vi "_Remote Prepare Mass Range.vi"(9 "Run Mode":T1, 10 "Fixed Mass (amu)":dbl, 11 "GUI Mass Ranges":T5[](array[typedef]) {"Res" items=["High/High", "Medium/Medium", "Low/Low", "High/Medium", "High/Low", "Medium/High", "Medium/Low", "Low/High", "Low/Medium"]}) -> (0 "Steps":i32[](array[numeric]), 1 "Dwell (ms)":dbl[](array[numeric]), 2 "Mass":dbl[](array[numeric]), 3 "Cycle Time (ms)":dbl, 4 "Init Q2 Mass":i32, 6 "Init Q1 Mass":i32, 7 "RT Mass Ranges":T2[](array[typedef]) {"Resolution Type" items=["High/High", "Medium/Medium", "Low/Low", "High/Medium", "High/Low", "Medium/High", "Medium/Low", "Low/High", "Low/Medium"]})   [LabVIEW 2015]
uses:
  Type/_Mass Range Property.ctl
  Type/_Mass Range Parameters.ctl
  Type/_RT Res Type.ctl
  Type/_RT Mass Range.ctl
  Type/_RT Active Ch.ctl
  Type/_Run Mode.ctl
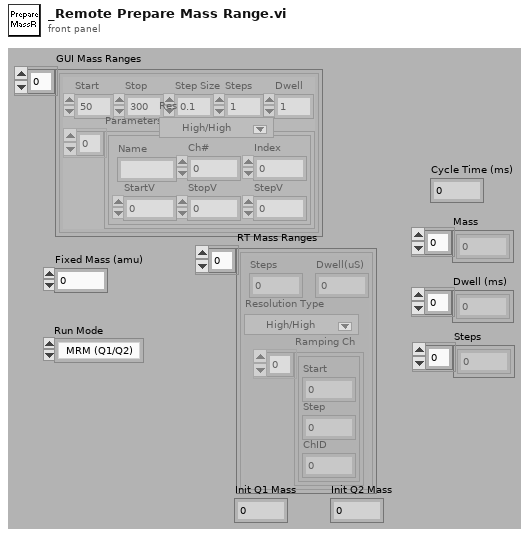
[diagram p1: front panel]
types:
  T1 = typedef "_Run Mode.ctl" = enum16{"MRM (Q1/Q2)", "Q1 Scan", "Q1 SRM", "Q2 Scan", "Q2 SRM", "Product Scan", "Precursor Scan", "Neutral Loss", "Neutral Gain"}
  T2 = typedef "_RT Mass Range.ctl" = cluster{"Steps":i32, "Dwell(uS)":i32, "Resolution Type":T3, "Ramping Ch":T4[]}
  T3 = typedef "_RT Res Type.ctl" = u16
  T4 = typedef "_RT Active Ch.ctl" = cluster{"Start":i32, "Step":i32, "ChID":i32}
  T5 = typedef "_Mass Range Property.ctl" = cluster{"Start":dbl, "Stop":dbl, "Step Size":dbl, "Steps":i32, "Dwell":dbl, "Parameters":T6[], "Res":T3}
  T6 = typedef "_Mass Range Parameters.ctl" = cluster{"Name":string, "Ch#":u8, "StartV":dbl, "StopV":dbl, "StepV":dbl, "Index":u8}
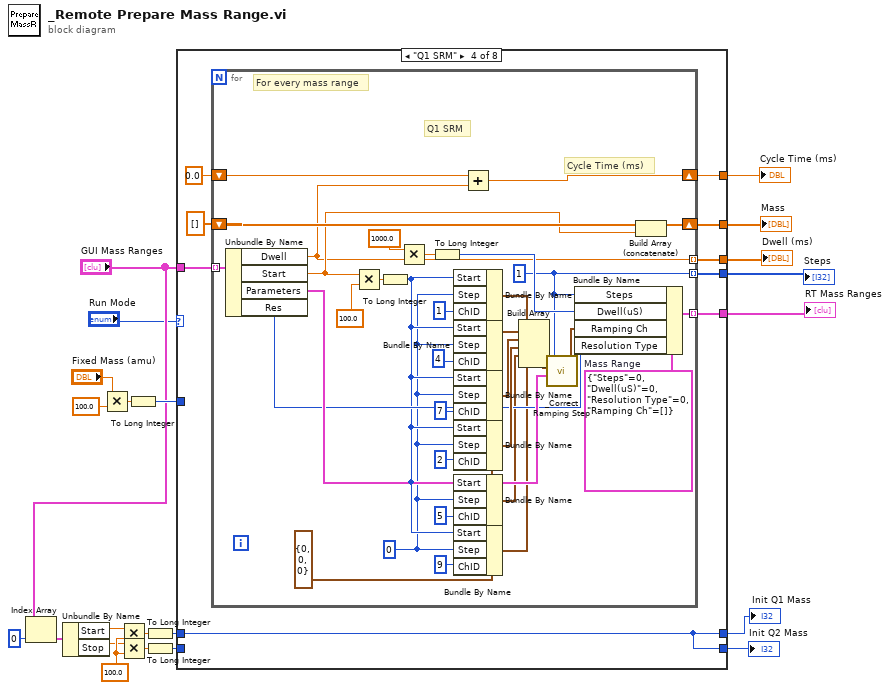
[diagram p0: block diagram]
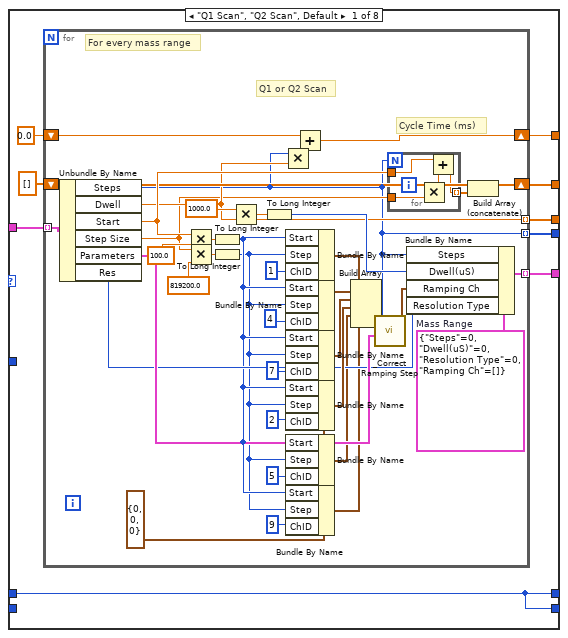
[diagram p2: hidden frame]
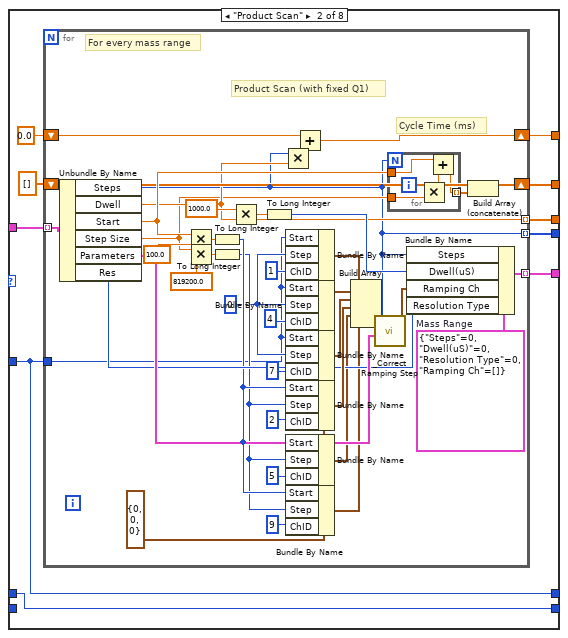
[diagram p3: hidden frame]
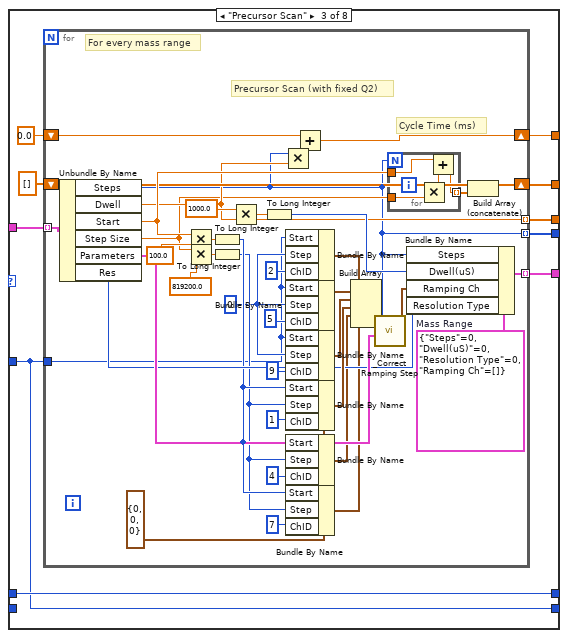
[diagram p4: hidden frame]
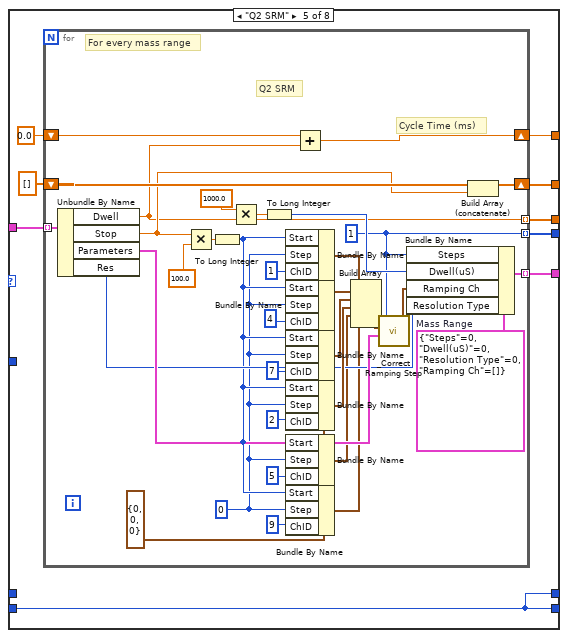
[diagram p5: hidden frame]
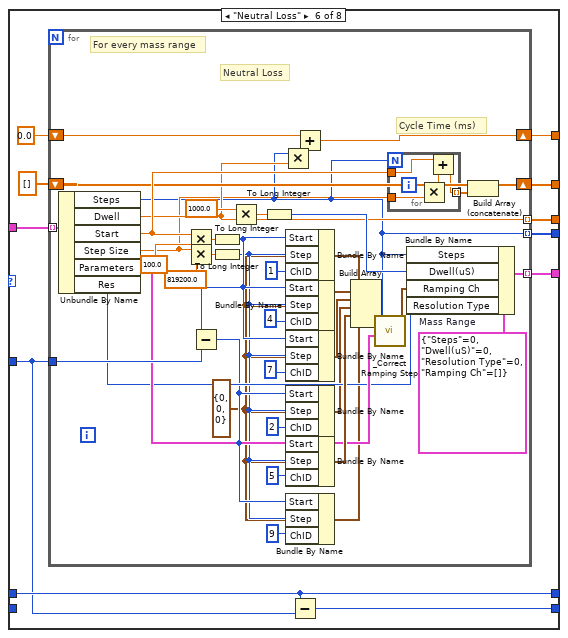
[diagram p6: hidden frame]
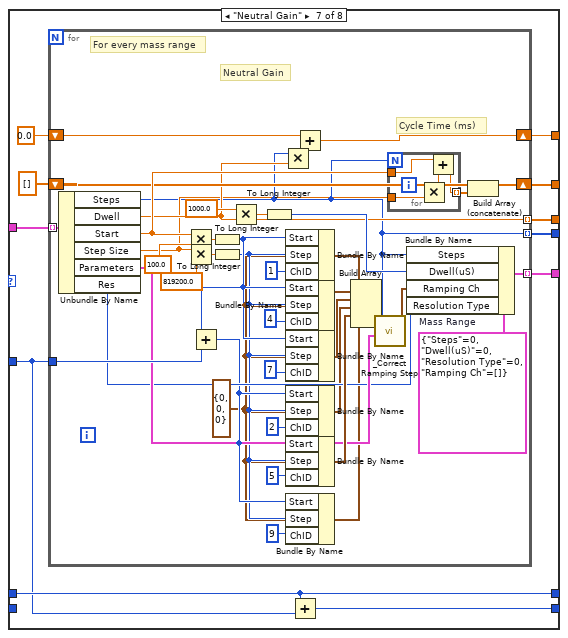
[diagram p7: hidden frame]
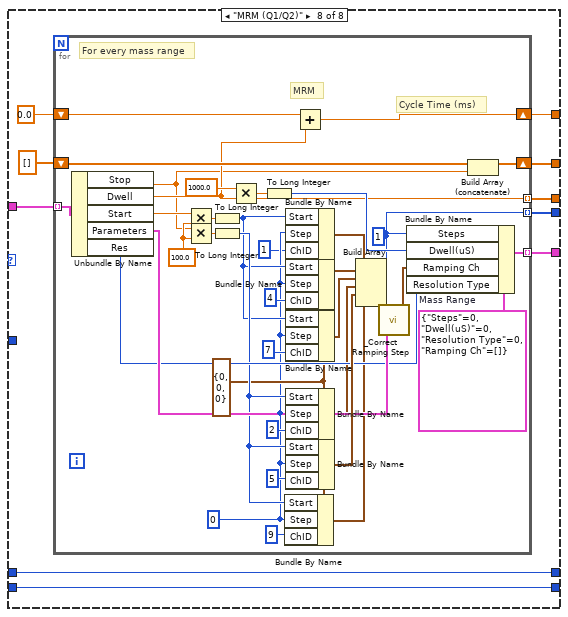
[diagram p8: hidden frame]
diagram:
  w8 = 100.0 ("y")
  n1 = Index Array(array="GUI Mass Ranges", index=0) -> (element=w11:T5)
  n2 = Unbundle By Name(w11) -> ("Start"=w7:dbl, "Stop"=w6:dbl)
  n3 = Multiply(x="Fixed Mass (amu)", y=100.0) -> (x*y=w17:dbl)
  n4 = Multiply(x=w7, y=w8) -> (x*y=w9:dbl)
  n5 = Multiply(x=w6, y=w8) -> (x*y=w10:dbl)
  n6 = To Long Integer(number=w17) -> (32bit integer=w14:i32)
  n7 = To Long Integer(number=w9) -> (32bit integer=w5:i32)
  n8 = To Long Integer(number=w10) -> (32bit integer=w4:i32)
  n9 = case shown="\"Q1 SRM\"" "Run Mode" {
    tunnel: "GUI Mass Ranges" -> [w31 w85 w141 w196 w239 w284 w341 w397]
    tunnel: [w30 w84 w140 w195 w238 w283 w340 w396] -> w22
    tunnel: [w29 w83 w139 w194 w237 w282 w339 w395] -> w21
    tunnel: [w28 w82 w138 w193 w236 w281 w338 w394] -> w20
    tunnel: [w27 w81 w137 w192 w235 w280 w337 w393] -> w19
    tunnel: [w26 w80 w136 w191 w234 w279 w336 w392] -> w18
    tunnel: w14 -> [_ w76 w132 _ _ w275 w332 _]
    tunnel: w5 -> [w23 w77 w133 w188 _ w276 w333 w389]
    tunnel: w4 -> [_ _ _ _ w231 _ _ w388]
    tunnel: [w23 w76 w133 w188 w231 w276 w333 w389] -> w3
    tunnel: [w23 w77 w132 w188 w231 w274 w331 w388] -> w2
    frame "Q1 Scan", "Q2 Scan", Default {
      n10 = for {
        tunnel: w31 -> [w70] mode=indexing
        tunnel: [w62] -> w26 mode=indexing
        shift-right: [w60] -> w30
        shift-left: 0.0 -> [w59]
        tunnel: [w41] -> w27 mode=indexing
        shift-right: [w55] -> w29
        shift-left: dbl[] [] -> [w56]
        tunnel: [w54] -> w28 mode=indexing
        w53 = T2 {"Steps"=0, "Dwell(uS)"=0, "Resolution Type"=0, "Ramping Ch"=[]}  # Mass Range
        w37 = T4 {"Start"=0, "Step"=0, "ChID"=0} ("Active Channel")
        # "Q1 or Q2 Scan"
        # "Cycle Time (ms)"
        # "For every mass range"
        n11 = Unbundle By Name(w70) -> ("Steps"=w41:i32, "Dwell"=w54:dbl, "Start"=w58:dbl, "Step Size"=w43:dbl, "Parameters"=w42:T6[], "Res"=w40:T3)
        n12 = Multiply(x=w58, y=100.0) -> (x*y=w68:dbl)
        n13 = Multiply(x=w43, y=819200.0) -> (x*y=w69:dbl)
        n14 = To Long Integer(number=w68) -> (32bit integer=w34:i32)
        n15 = To Long Integer(number=w69) -> (32bit integer=w33:i32)
        n16 = Multiply(x=1000.0, y=w54) -> (x*y=w64:dbl)
        n17 = To Long Integer(number=w64) -> (32bit integer=w63:i32)
        n18 = Multiply(x=w41, y=w54) -> (x*y=w61:dbl)
        n19 = Bundle By Name(cluster=w37, "Start"=w34, "Step"=w33, "ChID"=1) -> (w66:T4)
        n20 = Bundle By Name(cluster=w37, "Start"=w34, "Step"=w33, "ChID"=4) -> (w49:T4)
        n21 = Bundle By Name(cluster=w37, "Start"=w34, "Step"=w33, "ChID"=7) -> (w48:T4)
        n22 = Bundle By Name(cluster=w37, "Start"=w34, "Step"=w33, "ChID"=2) -> (w50:T4)
        n23 = Bundle By Name(cluster=w37, "Start"=w34, "Step"=w33, "ChID"=5) -> (w36:T4)
        n24 = Bundle By Name(cluster=w37, "Start"=w34, "Step"=w33, "ChID"=9) -> (w35:T4)
        n25 = Add(x=w59, y=w61) -> (x+y=w60:dbl)
        n26 = Build Array(w66, w49, w48, w50, w36, w35) -> (w52:T4[])
        n27 = call "_Correct Ramping Step.vi"("MR Parameters"=w42, "Ramping Masses"=w52, "Primary Steps"=w41) -> ("Ramping Channels"=w51:T4[])  [unwired: 4 out]
        n28 = for {
          N: w41 -> [_]
          tunnel: w43 -> [w74]
          tunnel: w58 -> [w72]
          tunnel: [w71] -> w57 mode=indexing
          i -> [w75]
          n29 = Multiply(x=w75, y=w74) -> (x*y=w73:dbl)
          n30 = Add(x=w72, y=w73) -> (x+y=w71:dbl)
        }
        n31 = Bundle By Name(cluster=w53, "Steps"=w41, "Dwell(uS)"=w63, "Ramping Ch"=w51, "Resolution Type"=w40) -> (w62:T2)
        n32 = Build Array (concatenate)(w56, w57) -> (w55:dbl[])
      }
    }
    frame "Product Scan" {
      n33 = for {
        tunnel: w85 -> [w126] mode=indexing
        tunnel: [w118] -> w80 mode=indexing
        shift-right: [w116] -> w84
        shift-left: 0.0 -> [w115]
        tunnel: [w97] -> w81 mode=indexing
        shift-right: [w111] -> w83
        shift-left: dbl[] [] -> [w112]
        tunnel: [w110] -> w82 mode=indexing
        tunnel: w76 -> [w87]
        w88 = 0 ("ChID")
        w109 = T2 {"Steps"=0, "Dwell(uS)"=0, "Resolution Type"=0, "Ramping Ch"=[]}  # Mass Range
        w93 = T4 {"Start"=0, "Step"=0, "ChID"=0} ("Active Channel")
        # "Product Scan (with fixed Q1)"
        # "Cycle Time (ms)"
        # "For every mass range"
        n34 = Unbundle By Name(w126) -> ("Steps"=w97:i32, "Dwell"=w110:dbl, "Start"=w114:dbl, "Step Size"=w99:dbl, "Parameters"=w98:T6[], "Res"=w96:T3)
        n35 = Multiply(x=w114, y=100.0) -> (x*y=w124:dbl)
        n36 = Multiply(x=w99, y=819200.0) -> (x*y=w125:dbl)
        n37 = To Long Integer(number=w124) -> (32bit integer=w90:i32)
        n38 = To Long Integer(number=w125) -> (32bit integer=w89:i32)
        n39 = Multiply(x=1000.0, y=w110) -> (x*y=w120:dbl)
        n40 = To Long Integer(number=w120) -> (32bit integer=w119:i32)
        n41 = Multiply(x=w97, y=w110) -> (x*y=w117:dbl)
        n42 = Bundle By Name(cluster=w93, "Start"=w87, "Step"=w88, "ChID"=1) -> (w122:T4)
        n43 = Bundle By Name(cluster=w93, "Start"=w87, "Step"=w88, "ChID"=4) -> (w105:T4)
        n44 = Bundle By Name(cluster=w93, "Start"=w87, "Step"=w88, "ChID"=7) -> (w104:T4)
        n45 = Bundle By Name(cluster=w93, "Start"=w90, "Step"=w89, "ChID"=2) -> (w106:T4)
        n46 = Bundle By Name(cluster=w93, "Start"=w90, "Step"=w89, "ChID"=5) -> (w92:T4)
        n47 = Bundle By Name(cluster=w93, "Start"=w90, "Step"=w89, "ChID"=9) -> (w91:T4)
        n48 = Add(x=w115, y=w117) -> (x+y=w116:dbl)
        n49 = Build Array(w122, w105, w104, w106, w92, w91) -> (w108:T4[])
        n50 = call "_Correct Ramping Step.vi"("MR Parameters"=w98, "Ramping Masses"=w108, "Primary Steps"=w97) -> ("Ramping Channels"=w107:T4[])  [unwired: 4 out]
        n51 = for {
          N: w97 -> [_]
          tunnel: w99 -> [w130]
          tunnel: w114 -> [w128]
          tunnel: [w127] -> w113 mode=indexing
          i -> [w131]
          n52 = Multiply(x=w131, y=w130) -> (x*y=w129:dbl)
          n53 = Add(x=w128, y=w129) -> (x+y=w127:dbl)
        }
        n54 = Bundle By Name(cluster=w109, "Steps"=w97, "Dwell(uS)"=w119, "Ramping Ch"=w107, "Resolution Type"=w96) -> (w118:T2)
        n55 = Build Array (concatenate)(w112, w113) -> (w111:dbl[])
      }
    }
    frame "Precursor Scan" {
      n56 = for {
        tunnel: w141 -> [w182] mode=indexing
        tunnel: [w174] -> w136 mode=indexing
        shift-right: [w172] -> w140
        shift-left: 0.0 -> [w171]
        tunnel: [w153] -> w137 mode=indexing
        shift-right: [w167] -> w139
        shift-left: dbl[] [] -> [w168]
        tunnel: [w166] -> w138 mode=indexing
        tunnel: w132 -> [w143]
        w144 = 0 ("ChID")
        w165 = T2 {"Steps"=0, "Dwell(uS)"=0, "Resolution Type"=0, "Ramping Ch"=[]}  # Mass Range
        w149 = T4 {"Start"=0, "Step"=0, "ChID"=0} ("Active Channel")
        # "Precursor Scan (with fixed Q2)"
        # "Cycle Time (ms)"
        # "For every mass range"
        n57 = Unbundle By Name(w182) -> ("Steps"=w153:i32, "Dwell"=w166:dbl, "Start"=w170:dbl, "Step Size"=w155:dbl, "Parameters"=w154:T6[], "Res"=w152:T3)
        n58 = Multiply(x=w170, y=100.0) -> (x*y=w180:dbl)
        n59 = Multiply(x=w155, y=819200.0) -> (x*y=w181:dbl)
        n60 = To Long Integer(number=w180) -> (32bit integer=w146:i32)
        n61 = To Long Integer(number=w181) -> (32bit integer=w145:i32)
        n62 = Multiply(x=1000.0, y=w166) -> (x*y=w176:dbl)
        n63 = To Long Integer(number=w176) -> (32bit integer=w175:i32)
        n64 = Multiply(x=w153, y=w166) -> (x*y=w173:dbl)
        n65 = Bundle By Name(cluster=w149, "Start"=w143, "Step"=w144, "ChID"=2) -> (w178:T4)
        n66 = Bundle By Name(cluster=w149, "Start"=w143, "Step"=w144, "ChID"=5) -> (w161:T4)
        n67 = Bundle By Name(cluster=w149, "Start"=w143, "Step"=w144, "ChID"=9) -> (w160:T4)
        n68 = Bundle By Name(cluster=w149, "Start"=w146, "Step"=w145, "ChID"=1) -> (w162:T4)
        n69 = Bundle By Name(cluster=w149, "Start"=w146, "Step"=w145, "ChID"=4) -> (w148:T4)
        n70 = Bundle By Name(cluster=w149, "Start"=w146, "Step"=w145, "ChID"=7) -> (w147:T4)
        n71 = Add(x=w171, y=w173) -> (x+y=w172:dbl)
        n72 = Build Array(w178, w161, w160, w162, w148, w147) -> (w164:T4[])
        n73 = call "_Correct Ramping Step.vi"("MR Parameters"=w154, "Ramping Masses"=w164, "Primary Steps"=w153) -> ("Ramping Channels"=w163:T4[])  [unwired: 4 out]
        n74 = for {
          N: w153 -> [_]
          tunnel: w155 -> [w186]
          tunnel: w170 -> [w184]
          tunnel: [w183] -> w169 mode=indexing
          i -> [w187]
          n75 = Multiply(x=w187, y=w186) -> (x*y=w185:dbl)
          n76 = Add(x=w184, y=w185) -> (x+y=w183:dbl)
        }
        n77 = Bundle By Name(cluster=w165, "Steps"=w153, "Dwell(uS)"=w175, "Ramping Ch"=w163, "Resolution Type"=w152) -> (w174:T2)
        n78 = Build Array (concatenate)(w168, w169) -> (w167:dbl[])
      }
    }
    frame "Q1 SRM" {
      n79 = for {
        tunnel: w196 -> [w230] mode=indexing
        tunnel: [w223] -> w191 mode=indexing
        shift-right: [w222] -> w195
        shift-left: 0.0 -> [w221]
        tunnel: [w199] -> w192 mode=indexing
        shift-right: [w219] -> w194
        shift-left: dbl[] [] -> [w220]
        tunnel: [w197] -> w193 mode=indexing
        w199 = 1 ("ChID")
        w200 = 0 ("ChID")
        w218 = T2 {"Steps"=0, "Dwell(uS)"=0, "Resolution Type"=0, "Ramping Ch"=[]}  # Mass Range
        w204 = T4 {"Start"=0, "Step"=0, "ChID"=0} ("Active Channel")
        # "Q1 SRM"
        # "Cycle Time (ms)"
        # "For every mass range"
        n80 = Unbundle By Name(w230) -> ("Dwell"=w197:dbl, "Start"=w198:dbl, "Parameters"=w208:T6[], "Res"=w207:T3)
        n81 = Multiply(x=w198, y=100.0) -> (x*y=w229:dbl)
        n82 = To Long Integer(number=w229) -> (32bit integer=w201:i32)
        n83 = Multiply(x=1000.0, y=w197) -> (x*y=w225:dbl)
        n84 = To Long Integer(number=w225) -> (32bit integer=w224:i32)
        n85 = Bundle By Name(cluster=w204, "Start"=w201, "Step"=w200, "ChID"=1) -> (w227:T4)
        n86 = Bundle By Name(cluster=w204, "Start"=w201, "Step"=w200, "ChID"=4) -> (w214:T4)
        n87 = Bundle By Name(cluster=w204, "Start"=w201, "Step"=w200, "ChID"=7) -> (w213:T4)
        n88 = Bundle By Name(cluster=w204, "Start"=w201, "Step"=w200, "ChID"=2) -> (w215:T4)
        n89 = Bundle By Name(cluster=w204, "Start"=w201, "Step"=w200, "ChID"=5) -> (w203:T4)
        n90 = Bundle By Name(cluster=w204, "Start"=w201, "Step"=w200, "ChID"=9) -> (w202:T4)
        n91 = Add(x=w221, y=w197) -> (x+y=w222:dbl)
        n92 = Build Array(w227, w214, w213, w215, w203, w202) -> (w217:T4[])
        n93 = call "_Correct Ramping Step.vi"("MR Parameters"=w208, "Ramping Masses"=w217, "Primary Steps"=w199) -> ("Ramping Channels"=w216:T4[])  [unwired: 4 out]
        n94 = Bundle By Name(cluster=w218, "Steps"=w199, "Dwell(uS)"=w224, "Ramping Ch"=w216, "Resolution Type"=w207) -> (w223:T2)
        n95 = Build Array (concatenate)(w220, w198) -> (w219:dbl[])
      }
    }
    frame "Q2 SRM" {
      n96 = for {
        tunnel: w239 -> [w273] mode=indexing
        tunnel: [w266] -> w234 mode=indexing
        shift-right: [w265] -> w238
        shift-left: 0.0 -> [w264]
        tunnel: [w242] -> w235 mode=indexing
        shift-right: [w262] -> w237
        shift-left: dbl[] [] -> [w263]
        tunnel: [w240] -> w236 mode=indexing
        w242 = 1 ("ChID")
        w243 = 0 ("ChID")
        w261 = T2 {"Steps"=0, "Dwell(uS)"=0, "Resolution Type"=0, "Ramping Ch"=[]}  # Mass Range
        w247 = T4 {"Start"=0, "Step"=0, "ChID"=0} ("Active Channel")
        # "Q2 SRM"
        # "Cycle Time (ms)"
        # "For every mass range"
        n97 = Unbundle By Name(w273) -> ("Dwell"=w240:dbl, "Stop"=w241:dbl, "Parameters"=w251:T6[], "Res"=w250:T3)
        n98 = Multiply(x=w241, y=100.0) -> (x*y=w272:dbl)
        n99 = To Long Integer(number=w272) -> (32bit integer=w244:i32)
        n100 = Multiply(x=1000.0, y=w240) -> (x*y=w268:dbl)
        n101 = To Long Integer(number=w268) -> (32bit integer=w267:i32)
        n102 = Bundle By Name(cluster=w247, "Start"=w244, "Step"=w243, "ChID"=1) -> (w270:T4)
        n103 = Bundle By Name(cluster=w247, "Start"=w244, "Step"=w243, "ChID"=4) -> (w257:T4)
        n104 = Bundle By Name(cluster=w247, "Start"=w244, "Step"=w243, "ChID"=7) -> (w256:T4)
        n105 = Bundle By Name(cluster=w247, "Start"=w244, "Step"=w243, "ChID"=2) -> (w258:T4)
        n106 = Bundle By Name(cluster=w247, "Start"=w244, "Step"=w243, "ChID"=5) -> (w246:T4)
        n107 = Bundle By Name(cluster=w247, "Start"=w244, "Step"=w243, "ChID"=9) -> (w245:T4)
        n108 = Add(x=w264, y=w240) -> (x+y=w265:dbl)
        n109 = Build Array(w270, w257, w256, w258, w246, w245) -> (w260:T4[])
        n110 = call "_Correct Ramping Step.vi"("MR Parameters"=w251, "Ramping Masses"=w260, "Primary Steps"=w242) -> ("Ramping Channels"=w259:T4[])  [unwired: 4 out]
        n111 = Bundle By Name(cluster=w261, "Steps"=w242, "Dwell(uS)"=w267, "Ramping Ch"=w259, "Resolution Type"=w250) -> (w266:T2)
        n112 = Build Array (concatenate)(w263, w241) -> (w262:dbl[])
      }
    }
    frame "Neutral Loss" {
      n113 = for {
        tunnel: w284 -> [w325] mode=indexing
        tunnel: [w318] -> w279 mode=indexing
        shift-right: [w316] -> w283
        shift-left: 0.0 -> [w315]
        tunnel: [w298] -> w280 mode=indexing
        shift-right: [w311] -> w282
        shift-left: dbl[] [] -> [w312]
        tunnel: [w310] -> w281 mode=indexing
        tunnel: w275 -> [w301]
        w309 = T2 {"Steps"=0, "Dwell(uS)"=0, "Resolution Type"=0, "Ramping Ch"=[]}  # Mass Range
        w289 = T4 {"Start"=0, "Step"=0, "ChID"=0} ("Active Channel")
        # "Neutral Loss"
        # "Cycle Time (ms)"
        # "For every mass range"
        n114 = Unbundle By Name(w325) -> ("Steps"=w298:i32, "Dwell"=w310:dbl, "Start"=w314:dbl, "Step Size"=w300:dbl, "Parameters"=w299:T6[], "Res"=w297:T3)
        n115 = Multiply(x=w314, y=100.0) -> (x*y=w323:dbl)
        n116 = Multiply(x=w300, y=819200.0) -> (x*y=w324:dbl)
        n117 = To Long Integer(number=w323) -> (32bit integer=w291:i32)
        n118 = Subtract(x=w291, y=w301) -> (x-y=w294:i32)
        n119 = To Long Integer(number=w324) -> (32bit integer=w290:i32)
        n120 = Multiply(x=1000.0, y=w310) -> (x*y=w320:dbl)
        n121 = To Long Integer(number=w320) -> (32bit integer=w319:i32)
        n122 = Multiply(x=w298, y=w310) -> (x*y=w317:dbl)
        n123 = Bundle By Name(cluster=w289, "Start"=w291, "Step"=w290, "ChID"=1) -> (w322:T4)
        n124 = Bundle By Name(cluster=w289, "Start"=w291, "Step"=w290, "ChID"=4) -> (w305:T4)
        n125 = Bundle By Name(cluster=w289, "Start"=w291, "Step"=w290, "ChID"=7) -> (w286:T4)
        n126 = Bundle By Name(cluster=w289, "Start"=w294, "Step"=w290, "ChID"=2) -> (w288:T4)
        n127 = Bundle By Name(cluster=w289, "Start"=w294, "Step"=w290, "ChID"=5) -> (w306:T4)
        n128 = Bundle By Name(cluster=w289, "Start"=w294, "Step"=w290, "ChID"=9) -> (w287:T4)
        n129 = Add(x=w315, y=w317) -> (x+y=w316:dbl)
        n130 = Build Array(w322, w305, w286, w288, w306, w287) -> (w308:T4[])
        n131 = call "_Correct Ramping Step.vi"("MR Parameters"=w299, "Ramping Masses"=w308, "Primary Steps"=w298) -> ("Ramping Channels"=w307:T4[])  [unwired: 4 out]
        n132 = for {
          N: w298 -> [_]
          tunnel: w300 -> [w329]
          tunnel: w314 -> [w327]
          tunnel: [w326] -> w313 mode=indexing
          i -> [w330]
          n133 = Multiply(x=w330, y=w329) -> (x*y=w328:dbl)
          n134 = Add(x=w327, y=w328) -> (x+y=w326:dbl)
        }
        n135 = Bundle By Name(cluster=w309, "Steps"=w298, "Dwell(uS)"=w319, "Ramping Ch"=w307, "Resolution Type"=w297) -> (w318:T2)
        n136 = Build Array (concatenate)(w312, w313) -> (w311:dbl[])
      }
      n137 = Subtract(x=w276, y=w275) -> (x-y=w274:i32)
    }
    frame "Neutral Gain" {
      n138 = for {
        tunnel: w341 -> [w382] mode=indexing
        tunnel: [w375] -> w336 mode=indexing
        shift-right: [w373] -> w340
        shift-left: 0.0 -> [w372]
        tunnel: [w355] -> w337 mode=indexing
        shift-right: [w368] -> w339
        shift-left: dbl[] [] -> [w369]
        tunnel: [w367] -> w338 mode=indexing
        tunnel: w332 -> [w358]
        w366 = T2 {"Steps"=0, "Dwell(uS)"=0, "Resolution Type"=0, "Ramping Ch"=[]}  # Mass Range
        w346 = T4 {"Start"=0, "Step"=0, "ChID"=0} ("Active Channel")
        # "Neutral Gain"
        # "Cycle Time (ms)"
        # "For every mass range"
        n139 = Unbundle By Name(w382) -> ("Steps"=w355:i32, "Dwell"=w367:dbl, "Start"=w371:dbl, "Step Size"=w357:dbl, "Parameters"=w356:T6[], "Res"=w354:T3)
        n140 = Multiply(x=w371, y=100.0) -> (x*y=w380:dbl)
        n141 = Multiply(x=w357, y=819200.0) -> (x*y=w381:dbl)
        n142 = To Long Integer(number=w380) -> (32bit integer=w348:i32)
        n143 = Add(x=w348, y=w358) -> (x+y=w351:i32)
        n144 = To Long Integer(number=w381) -> (32bit integer=w347:i32)
        n145 = Multiply(x=1000.0, y=w367) -> (x*y=w377:dbl)
        n146 = To Long Integer(number=w377) -> (32bit integer=w376:i32)
        n147 = Multiply(x=w355, y=w367) -> (x*y=w374:dbl)
        n148 = Bundle By Name(cluster=w346, "Start"=w348, "Step"=w347, "ChID"=1) -> (w379:T4)
        n149 = Bundle By Name(cluster=w346, "Start"=w348, "Step"=w347, "ChID"=4) -> (w362:T4)
        n150 = Bundle By Name(cluster=w346, "Start"=w348, "Step"=w347, "ChID"=7) -> (w343:T4)
        n151 = Bundle By Name(cluster=w346, "Start"=w351, "Step"=w347, "ChID"=2) -> (w345:T4)
        n152 = Bundle By Name(cluster=w346, "Start"=w351, "Step"=w347, "ChID"=5) -> (w363:T4)
        n153 = Bundle By Name(cluster=w346, "Start"=w351, "Step"=w347, "ChID"=9) -> (w344:T4)
        n154 = Add(x=w372, y=w374) -> (x+y=w373:dbl)
        n155 = Build Array(w379, w362, w343, w345, w363, w344) -> (w365:T4[])
        n156 = call "_Correct Ramping Step.vi"("MR Parameters"=w356, "Ramping Masses"=w365, "Primary Steps"=w355) -> ("Ramping Channels"=w364:T4[])  [unwired: 4 out]
        n157 = for {
          N: w355 -> [_]
          tunnel: w357 -> [w386]
          tunnel: w371 -> [w384]
          tunnel: [w383] -> w370 mode=indexing
          i -> [w387]
          n158 = Multiply(x=w387, y=w386) -> (x*y=w385:dbl)
          n159 = Add(x=w384, y=w385) -> (x+y=w383:dbl)
        }
        n160 = Bundle By Name(cluster=w366, "Steps"=w355, "Dwell(uS)"=w376, "Ramping Ch"=w364, "Resolution Type"=w354) -> (w375:T2)
        n161 = Build Array (concatenate)(w369, w370) -> (w368:dbl[])
      }
      n162 = Add(x=w333, y=w332) -> (x+y=w331:i32)
    }
    frame "MRM (Q1/Q2)" {
      n163 = for {
        tunnel: w397 -> [w434] mode=indexing
        tunnel: [w426] -> w392 mode=indexing
        shift-right: [w425] -> w396
        shift-left: 0.0 -> [w424]
        tunnel: [w414] -> w393 mode=indexing
        shift-right: [w422] -> w395
        shift-left: dbl[] [] -> [w423]
        tunnel: [w417] -> w394 mode=indexing
        w400 = 0 ("ChID")
        w414 = 1 ("Steps")
        w421 = T2 {"Steps"=0, "Dwell(uS)"=0, "Resolution Type"=0, "Ramping Ch"=[]}  # Mass Range
        w431 = 100.0 ("y")
        w403 = T4 {"Start"=0, "Step"=0, "ChID"=0} ("Active Channel")
        # "MRM"
        # "Cycle Time (ms)"
        # "For every mass range"
        n164 = Unbundle By Name(w434) -> ("Stop"=w398:dbl, "Dwell"=w417:dbl, "Start"=w416:dbl, "Parameters"=w413:T6[], "Res"=w411:T3)
        n165 = Multiply(x=w416, y=w431) -> (x*y=w432:dbl)
        n166 = Multiply(x=w398, y=w431) -> (x*y=w433:dbl)
        n167 = To Long Integer(number=w432) -> (32bit integer=w406:i32)
        n168 = To Long Integer(number=w433) -> (32bit integer=w408:i32)
        n169 = Multiply(x=1000.0, y=w417) -> (x*y=w428:dbl)
        n170 = To Long Integer(number=w428) -> (32bit integer=w427:i32)
        n171 = Bundle By Name(cluster=w403, "Start"=w408, "Step"=w400, "ChID"=9) -> (w404:T4)
        n172 = Bundle By Name(cluster=w403, "Start"=w406, "Step"=w400, "ChID"=1) -> (w430:T4)
        n173 = Bundle By Name(cluster=w403, "Start"=w406, "Step"=w400, "ChID"=4) -> (w419:T4)
        n174 = Bundle By Name(cluster=w403, "Start"=w406, "Step"=w400, "ChID"=7) -> (w401:T4)
        n175 = Bundle By Name(cluster=w403, "Start"=w408, "Step"=w400, "ChID"=2) -> (w402:T4)
        n176 = Bundle By Name(cluster=w403, "Start"=w408, "Step"=w400, "ChID"=5) -> (w420:T4)
        n177 = Add(x=w424, y=w417) -> (x+y=w425:dbl)
        n178 = Build Array(w430, w419, w401, w402, w420, w404) -> (w415:T4[])
        n179 = call "_Correct Ramping Step.vi"("MR Parameters"=w413, "Ramping Masses"=w415, "Primary Steps"=w414) -> ("Ramping Channels"=w412:T4[])  [unwired: 4 out]
        n180 = Bundle By Name(cluster=w421, "Steps"=w414, "Dwell(uS)"=w427, "Ramping Ch"=w412, "Resolution Type"=w411) -> (w426:T2)
        n181 = Build Array (concatenate)(w423, w398) -> (w422:dbl[])
      }
    }
  }
  "Cycle Time (ms)" <- w22
  "Mass" <- w21
  "Dwell (ms)" <- w20
  "Steps" <- w19
  "RT Mass Ranges" <- w18
  "Init Q2 Mass" <- w2
  "Init Q1 Mass" <- w3
